vi "parse_int16.vi"   [LabVIEW 2010]
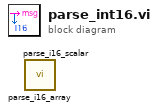
[diagram p0: block diagram]
diagram:
  n1 = call <userlib>:"parse_i16_array.vi"() -> ()  [unwired: 5 in, 3 out]
  n2 = call <userlib>:"parse_i16_scalar.vi"() -> ()  [unwired: 5 in, 3 out]
